vi "Lim_FileGetAttributes.vi"(8 "error in (no error)":errorcluster, 11 "hFile in":T3) -> (0 "error out":errorcluster, 1 "LIMRESULT":T1 items=["LIM_OK"=0, "LIM_ERR_UNEXPECTED"=-1, "LIM_ERR_NOTIMPL"=-2, "LIM_ERR_OUTOFMEMORY"=-3, "LIM_ERR_INVALIDARG "=-4, "LIM_ERR_NOINTERFACE"=-5, "LIM_ERR_POINTER"=-6, "LIM_ERR_FAIL"=-9, "LIM_ERR_NOTFOUND"=-13], 2 "LIMATTRIBUTES":T2, 3 "hFile out":T3, 5 "N Frames (uiSequenceCount)":u32)   [LabVIEW 2014, in "ND2_Reader_32.lvlib"]
uses:
  ND2_Reader_32.lvlib
  controls/numeric_LIMFILEHANDLE.ctl
  controls/cluster_LIMATTRIBUTES.ctl
  controls/numeric_LIMRESULT.ctl
  nd2 reader/SDK/bin/x86/v6_w32_nd2ReadSDK.dll
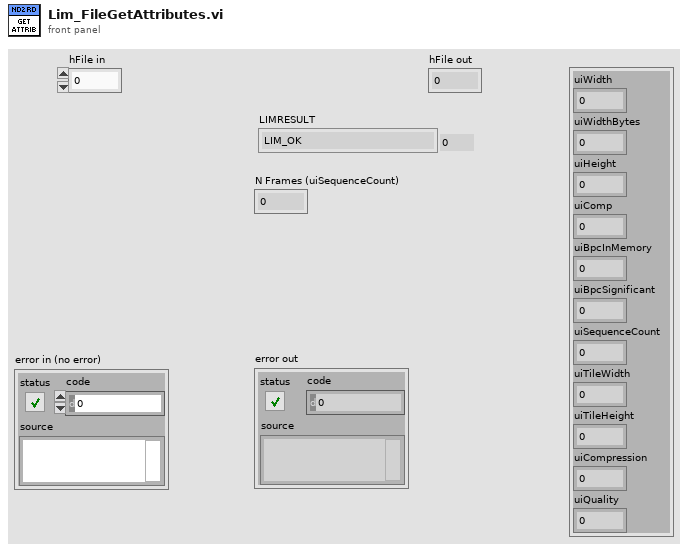
[diagram p1: front panel]
types:
  T1 = typedef "numeric_LIMRESULT.ctl" = i32
  T2 = typedef "cluster_LIMATTRIBUTES.ctl" = cluster{"uiWidth":u32, "uiWidthBytes":u32, "uiHeight":u32, "uiComp":u32, "uiBpcInMemory":u32, "uiBpcSignificant":u32, "uiSequenceCount":u32, "uiTileWidth":u32, "uiTileHeight":u32, "uiCompression":u32, "uiQuality":u16}
  T3 = typedef "numeric_LIMFILEHANDLE.ctl" = i32
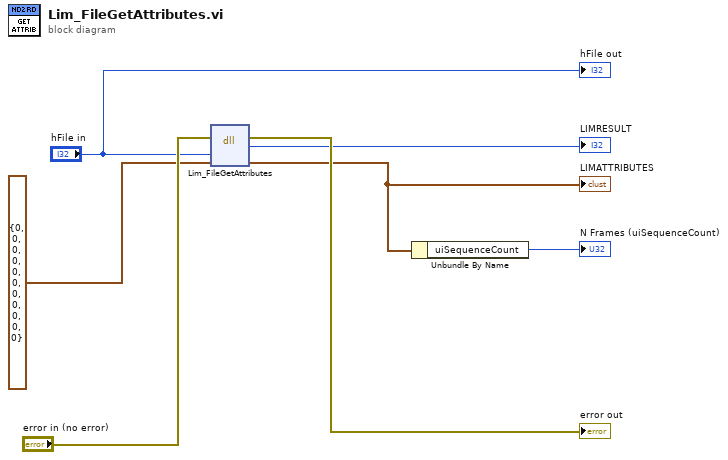
[diagram p0: block diagram]
diagram:
  n1 = dll-call lib="C:/Users/VirtualUser/Desktop/EPA-Vision/EPA Image Source LV2014 2.0.0 2016-02-23/ND2_Reader_32bit/nd2 reader/SDK/bin/x86/v6_w32_nd2ReadSDK.dll" fn="Lim_FileGetAttributes"(error in="error in (no error)", "hfile"="hFile in", "pFileAttributes"=T2 {"uiWidth"=0, "uiWidthBytes"=0, "uiHeight"=0, "uiComp"=0, "uiBpcInMemory"=0, "uiBpcSignificant"=0, "uiSequenceCount"=0, "uiTileWidth"=0, "uiTileHeight"=0, "uiCompression"=0, "uiQuality"=0} ("LIMATTRIBUTES")) -> (error out=→"error out":errorcluster, "LIMRESULT"=→"LIMRESULT":i32, "pFileAttributes"=w2:T2)  [unwired: 2 in, 2 out]
  "LIMATTRIBUTES" <- w2
  n2 = Unbundle By Name(w2) -> ("uiSequenceCount"=→"N Frames (uiSequenceCount)":u32)
  "hFile out" <- "hFile in"
